vi "APS get trigger fifo status.vi"(8 "error in (no error)":errorcluster caption="错误输入（无错误）", 9 "FifoSts":i32, 10 "FCmpCh":i32, 11 "Board_ID":i32) -> (0 "error out":errorcluster caption="错误输出", 1 "FifoSts out":i32, 3 "function return":i32)   [LabVIEW 2011, in "APS168.lvlib"]
doc: "I32 FNTYPE APS_get_trigger_fifo_status( I32 Board_ID, I32 FCmpCh, I32 *FifoSts );"
uses:
  APS168.lvlib
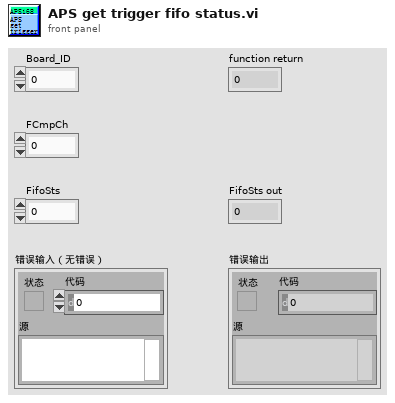
[diagram p1: front panel]
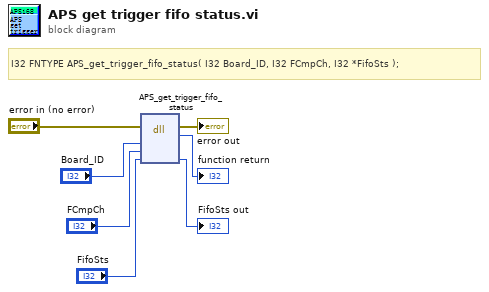
[diagram p0: block diagram]
diagram:
  # "I32 FNTYPE APS_get_trigger_fifo_status( I32 Board_ID, I32 FCmpCh, I32 *FifoSts );"
  n1 = dll-call lib="PTH1Labs E软件ADLINK 204CAPS_1_7_1_LIB line 连续运动204APS168.*" fn="APS_get_trigger_fifo_status"(error in="error in (no error)", "Board_ID"="Board_ID", "FCmpCh"="FCmpCh", "FifoSts"="FifoSts") -> (error out=→"error out":errorcluster, →"function return":i32, "FifoSts"=→"FifoSts out":i32)  [unwired: 4 in, 1 out]
